vi "Get Channels Block Descriptor.vi"(8 "error in (no error)":errorcluster, 11 "Transfer Runtime in":refnum<class "Runtime.Transfer.lvclass">) -> (0 "error out":errorcluster, 2 "block descriptor":T1 {"size" format="%016x"; "pointer" format="%016x"}, 3 "Transfer Runtime out":refnum<class "Runtime.Transfer.lvclass">)   [LabVIEW 2016, in "Data Sharing Framework.Runtime.lvlib" / "Runtime.Transfer.lvclass"]
uses:
  Runtime.Transfer.lvclass
  Typedefs/Block Descriptor.ctl
  Runtime.Transfer.lvclass/Runtime.Transfer.ctl
  APIs/Runtime/Data Sharing Framework.Runtime.lvlib
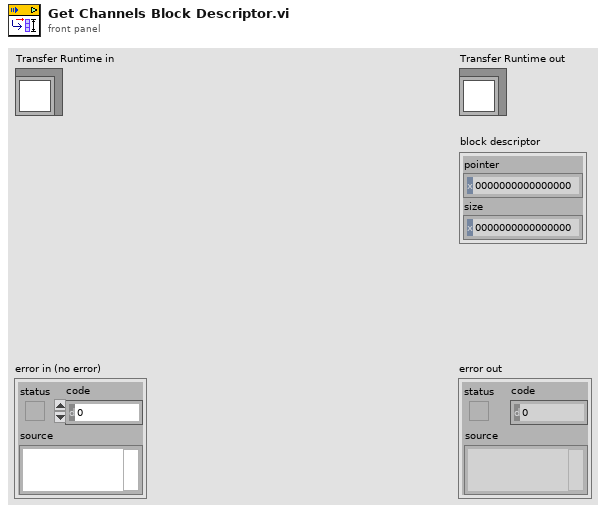
[diagram p1: front panel]
types:
  T1 = typedef "Data Sharing Framework.Runtime.lvlib/Block Descriptor.ctl" = cluster{"pointer":u64, "size":u64}
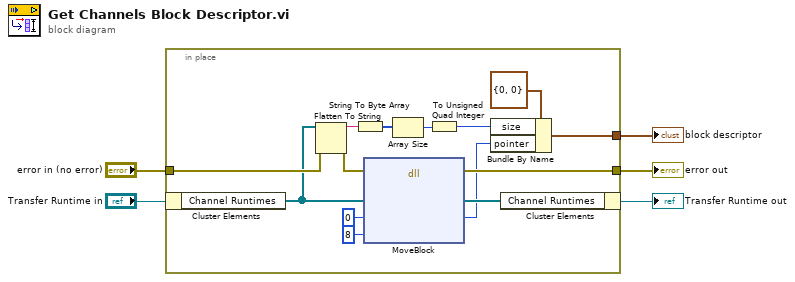
[diagram p0: block diagram]
diagram:
  n1 = in-place {
    in-place-border: "error in (no error)" -> [w15]
    in-place-border: [w17] -> w2
    in-place-border: [w6] -> w1
    n2 = in-place-cluster #1("Transfer Runtime in") -> ("Channel Runtimes"=w13:refnum<class "Runtime.Channel.lvclass">[])
    n3 = Flatten To String(anything=w13, error in (no error)=w15) -> (data string=w10:string, error out=w14:errorcluster)  [unwired: 2 in, 1 out]
    n4 = String To Byte Array(string=w10) -> (unsigned byte array=w9:u8[])
    n5 = dll-call lib="LabVIEW" fn="MoveBlock"(error in=w14, "src"=w13, "dst"=u64 0, "size"=8) -> (error out=w17:errorcluster, "src"=w19:refnum<class "Runtime.Channel.lvclass">[], "dst"=w11:u64)  [unwired: 4 in, 1 out]
    n6 = Array Size(array=w9) -> (size(s)=w8:i32)
    n7 = To Unsigned Quad Integer(1:w8) -> (0:w7:u64)
    n8 = Bundle By Name(cluster=T1 {"pointer"=0, "size"=0} ("block descriptor"), "size"=w7, "pointer"=w11) -> (w6:T1)
    n9 = in-place-cluster #1("Channel Runtimes"=w19) -> (→"Transfer Runtime out":refnum<class "Runtime.Transfer.lvclass">)
  }
  "error out" <- w2
  "block descriptor" <- w1
